vi "Condition jsObject.vi"(7 "Connection Refnum":T1, 8 "error in (no error)":errorcluster, 9 "Condition Record (empty)":T2, 10 "Condition jsObject Name (\"\")":string, 11 "Previous String (\"\")":string) -> (0 "error out":errorcluster, 2 "Condition jsObject":string, 3 "CONDITION jsObject Definition":string, 5 "dup Connection Refnum":T1)   [LabVIEW 2011]
uses:
  Condition Record.ctl
  Condition Operators.ctl
  SI.LIB/ODBC/SQL Controls/Connection Refnum.ctl
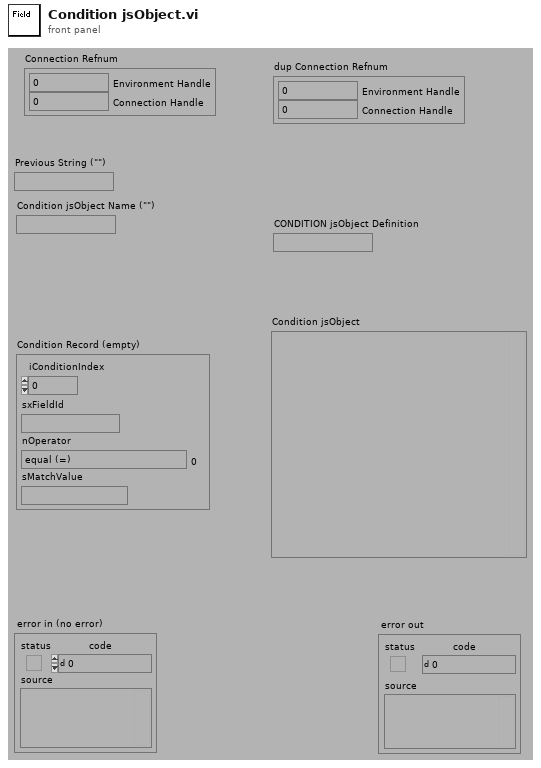
[diagram p1: front panel]
types:
  T1 = typedef "Connection Refnum.ctl" = cluster{"Environment Handle":i32, "Connection Handle":i32}
  T2 = typedef "Condition Record.ctl" = cluster{"iConditionIndex":i32, "sxFieldId":string, "nOperator":T3, "sMatchValue":string}
  T3 = typedef "Condition Operators.ctl" = enum16{"equal (=)", "not equal (\\u2260)", "less than (<)", "less than or equal (\\u2264)", "greater than (>)", "greater than or equal (\\u2265)", "contains", "does not contain"}
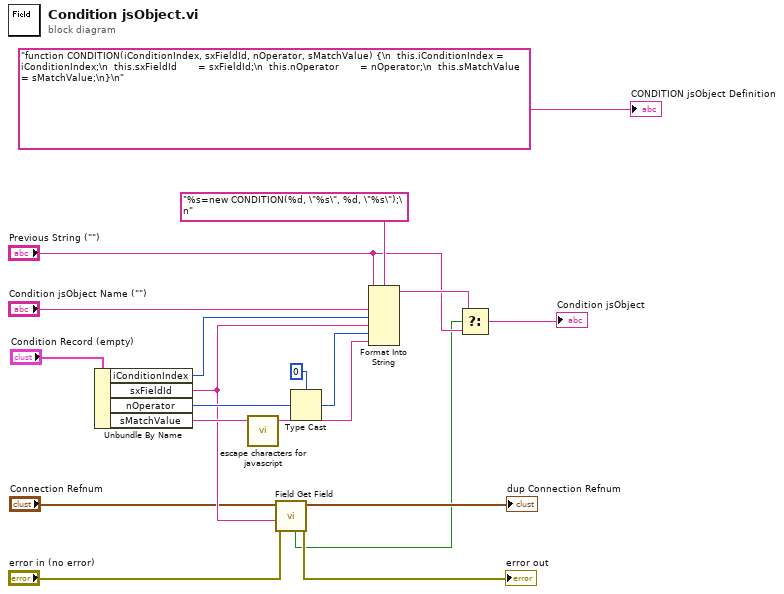
[diagram p0: block diagram]
diagram:
  n1 = Unbundle By Name("Condition Record (empty)") -> ("iConditionIndex"=w11:i32, "sxFieldId"=w9:string, "nOperator"=w16:T3, "sMatchValue"=w14:string)
  n2 = call "escape characters for javascript.vi"("String (\"\")"=w14) -> ("escaped String"=w10:string)  [unwired: 4 out]
  n3 = call "Field Get Field.vi"("error in (no error)"="error in (no error)", "sFieldId or sDisplayName (\"\")"=w9, "Connection Refnum"="Connection Refnum") -> ("error out"=→"error out":errorcluster, "Connection Refnum"=→"dup Connection Refnum":T1, "Data Present?"=w1:bool)  [unwired: 2 in, 4 out]
  n4 = Type Cast(type=u16 0, x=w16) -> (*(type *) &x=w15:u16)
  n5 = Format Into String(format string="%s=new CONDITION(%d, \"%s\", %d, \"%s\");\n", initial string="Previous String (\"\")", "Condition jsObject Name (\"\")", w11, w9, w15, w10) -> (resulting string=w4:string)  [unwired: 1 in, 1 out]
  n6 = Select(t=w4, s=w1, f="Previous String (\"\")") -> (s? t:f=→"Condition jsObject":string)
  "CONDITION jsObject Definition" <- "function CONDITION(iConditionIndex, sxFieldId, nOperator, sMatchValue) {\n  this.iConditionIndex = iConditionIndex;\n  this.sxFieldId       = sxFieldId;\n  this.nOperator       = nOperator;\n  this.sMatchValue     = sMatchValue;\n}\n"
